vi "ex4_1.vi"() -> ()   [LabVIEW 2019]
panel:
  in  "stop":bool
  out "Boolean":bool
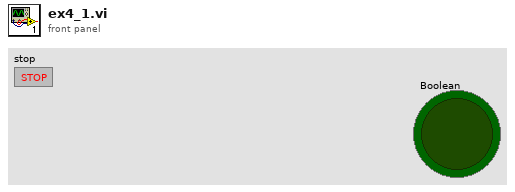
[diagram p1: front panel]
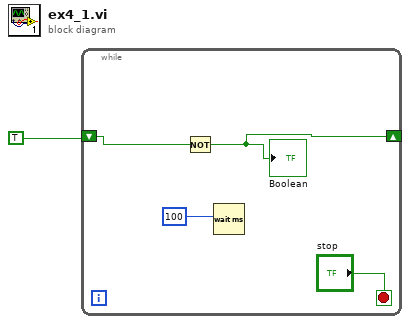
[diagram p0: block diagram]
diagram:
  n1 = while {
    shift-right: [w3] -> _
    shift-left: TRUE -> [w5]
    stop <- "stop" stop-if-true
    n2 = Not(x=w5) -> (.not. x?=w3:bool)
    "Boolean" <- w3
    n3 = Wait (ms)(milliseconds to wait=100) -> ()  [unwired: 1 out]
  }
